vi "Button_Click.vi"(0 "Button_1":bool caption="Button 1", 5 "Button_2":bool caption="Button 2", 11 "Error_In":errorcluster) -> (15 "Error_Out":errorcluster)   [LabVIEW 2023]
doc: "This VI alternatively Clicks two boolean buttons until key down happens,"
uses:
  Controls/Click_On.ctl
panel:
  # "."
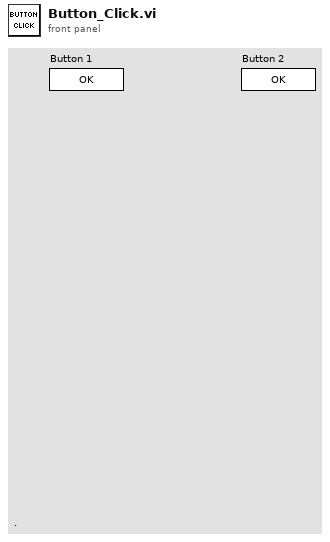
[diagram p1: front panel]
types:
  T1 = typedef "Click_On.ctl" = enum16{"Button 1", "Button 2"}
  T2 = typedef "LVRectTypeDef.ctl" = cluster{"Left":i16, "Top":i16, "Right":i16, "Bottom":i16}
  T3 = typedef "LVPositionTypeDef.ctl" = cluster{"Left":i32, "Top":i32}
  T4 = enum16{"Left Button", "Center Button", "Right Button", "Window Close"}
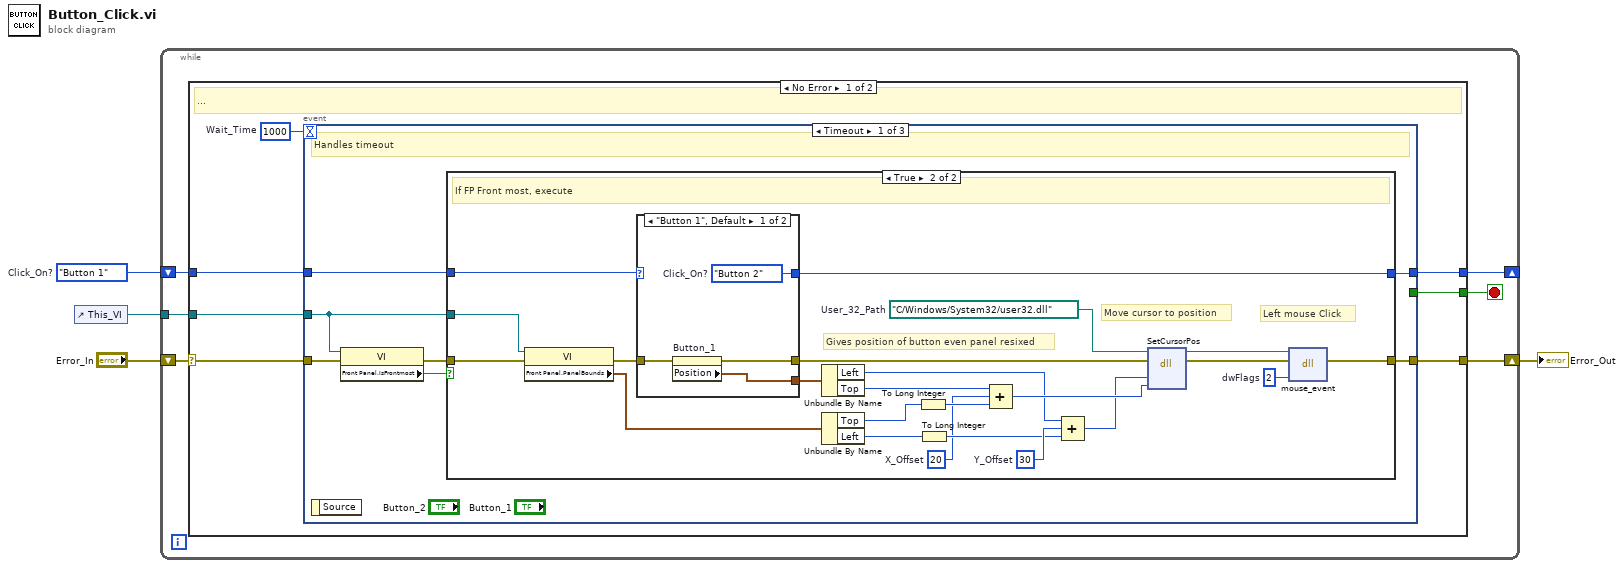
[diagram p0: block diagram]
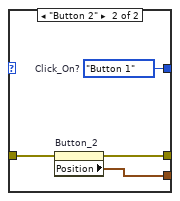
[diagram p3: hidden frame]
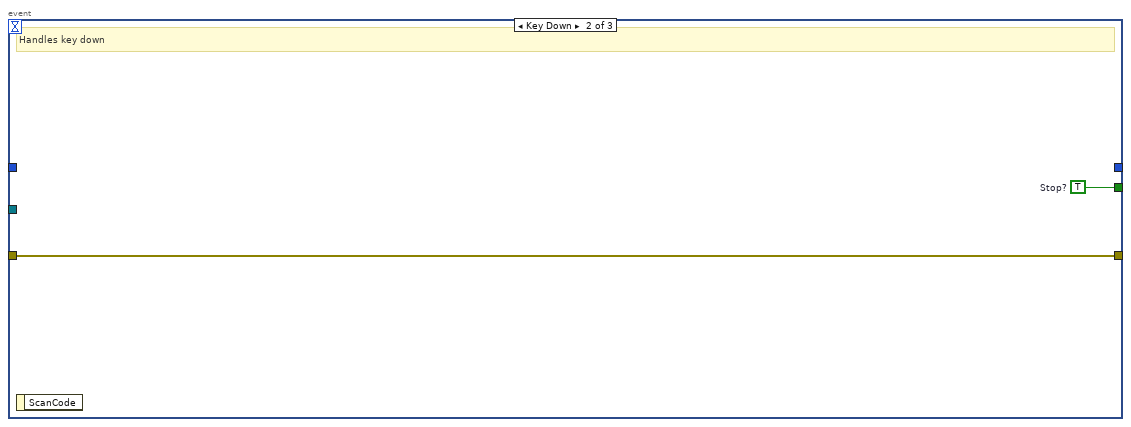
[diagram p4: hidden frame]
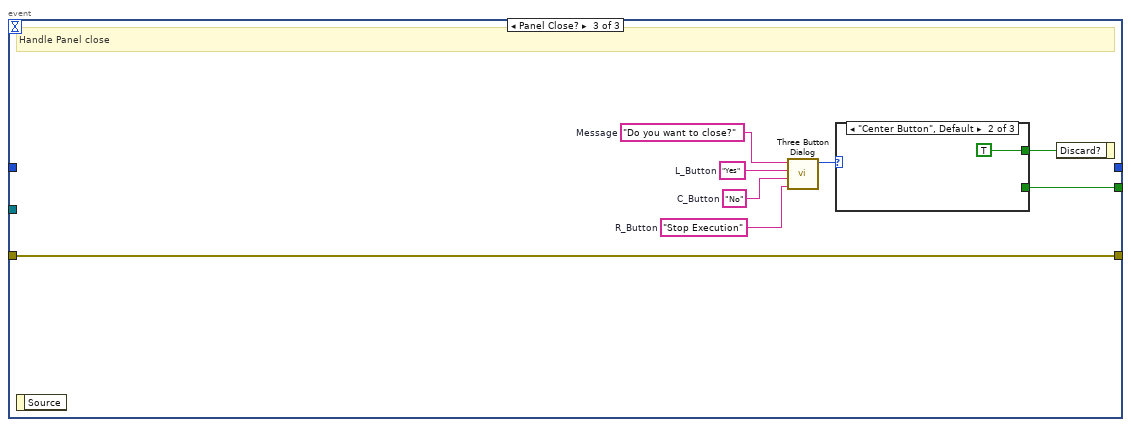
[diagram p5: hidden frame]
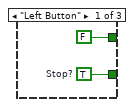
[diagram p6: hidden frame]
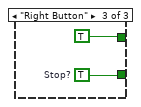
[diagram p7: hidden frame]
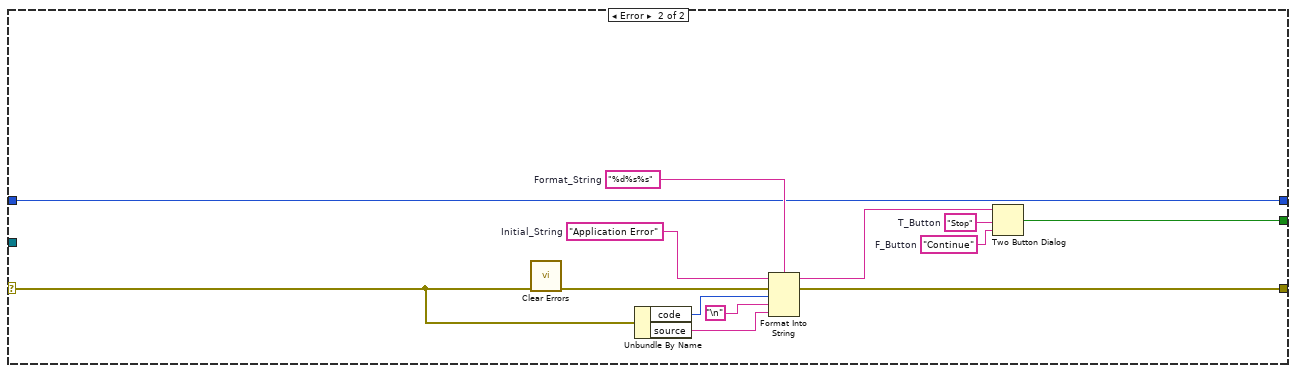
[diagram p8: hidden frame]
diagram:
  w3 = Click_On."Button 1"  # Click_On?
  n1 = control-ref of="This_VI"() -> (w1:refnum<vi>)
  n2 = while {
    shift-right: [w9] -> _
    shift-left: w3 -> [w7]
    shift-right: [w8] -> w4
    shift-left: "Error_In" -> [w10]
    tunnel: w1 -> [w5]
    stop <- w6 stop-if-true
    n3 = case shown="No Error" w10 {
      selector: w10 -> [w16 w73]
      tunnel: [w15 w74] -> w9
      tunnel: [w14 w76] -> w8
      tunnel: w7 -> [w13 w74]
      tunnel: [w12 w75] -> w6
      tunnel: w5 -> [w11 _]
      frame No Error {
        w17 = 1000  # Wait_Time
        # "..."
        n4 = event shown="[0] Timeout" {
          selector: _ -> [_ _ _]
          dyn-events: _ -> [_ _ _]
          timeout: w17 -> [_ _ _]
          tunnel: w16 -> [w21 w59 w61]
          tunnel: [w24 _ _] -> w15
          tunnel: [w22 w59 w61] -> w14
          tunnel: w13 -> [w23 _ _]
          tunnel: [_ w58 w62] -> w12
          tunnel: w11 -> [w19 _ _]
          event Timeout {
            # "Handles timeout"
            n5 = event-data() -> ()  [unwired: 1 in, 1 out]
            n6 = property class="VI"(reference=w19, error in=w21) -> (error out=w20:errorcluster, "Front Panel.IsFrontmost"=w18:bool)  [unwired: 1 out]
            n7 = case shown="True" w18 {
              tunnel: [w25 w49] -> w24
              tunnel: w23 -> [w25 w48]
              tunnel: [w26 w46] -> w22
              tunnel: w20 -> [w26 w39]
              tunnel: w19 -> [_ w30]
              frame False {
                # "If FP not front most, dont execute"
              }
              frame True {
                w28 = path "C:/Windows/System32/user32.dll"  # User_32_Path
                w45 = 2  # dwFlags
                w29 = 20  # X_Offset
                w43 = 30  # Y_Offset
                # "Gives position of button even panel resixed"
                # "Left mouse Click"
                # "Move cursor to position"
                # "If FP Front most, execute"
                n8 = property class="VI"(reference=w30, error in=w39) -> (error out=w38:errorcluster, "Front Panel.PanelBounds"=w31:T2)  [unwired: 1 out]
                n9 = case shown="\"Button 1\", Default" w48 {
                  tunnel: w38 -> [w53 w55]
                  tunnel: [w52 w57] -> w41
                  tunnel: [w51 w56] -> w40
                  tunnel: [w50 w54] -> w49
                  frame "Button 1", Default {
                    w50 = Click_On."Button 2"  # Click_On?
                    n10 = property on="Button_1" class="Bool (strict)"(error in=w53) -> (error out=w52:errorcluster, "Position"=w51:T3)  [unwired: 1 in, 1 out]
                  }
                  frame "Button 2" {
                    w54 = Click_On."Button 1"  # Click_On?
                    n11 = property on="Button_2" class="Bool (strict)"(error in=w55) -> (error out=w57:errorcluster, "Position"=w56:T3)  [unwired: 1 in, 1 out]
                  }
                }
                n12 = Unbundle By Name(w40) -> ("Left"=w37:i32, "Top"=w36:i32)
                n13 = Unbundle By Name(w31) -> ("Top"=w35:i16, "Left"=w33:i16)
                n14 = To Long Integer(number=w35) -> (32bit integer=w34:i32)
                n15 = To Long Integer(number=w33) -> (32bit integer=w32:i32)
                n16 = Compound Arithmetic op=ADD(w36, w29, w34) -> (w44:i32)
                n17 = Compound Arithmetic op=ADD(w37, w43, w32) -> (w42:i32)
                n18 = dll-call lib="?" fn="SetCursorPos"(path in=w28, error in=w41, "X_Coord"=w42, "Y_Coord"=w44) -> (path out=w27:path, error out=w47:errorcluster)  [unwired: 4 in]
                n19 = dll-call lib="?" fn="mouse_event"(path in=w27, error in=w47, "dwFlags"=w45) -> (error out=w46:errorcluster)  [unwired: 3 in, 1 out]
              }
            }
          }
          event Key Down {
            w58 = TRUE  # Stop?
            # "Handles key down"
            n20 = event-data() -> ()  [unwired: 1 in, 1 out]
          }
          event Panel Close? {
            w60 = "Stop Execution"  # R_Button
            w65 = "No"  # C_Button
            w66 = "Yes"  # L_Button
            w67 = "Do you want to close?"  # Message
            # "Handle Panel close"
            n21 = event-data() -> ()  [unwired: 1 in, 1 out]
            n22 = call <vilib>:"Three Button Dialog.vi"("Right Button Text (\"Cancel\")"=w60, "Center Button Text (\"No\")"=w65, "Left Button Text (\"Yes\")"=w66, "message"=w67) -> ("Which Button?"=w64:T4)  [unwired: 7 in]
            n23 = case shown="\"Center Button\", Default" w64 {
              tunnel: [FALSE TRUE TRUE] -> w63
              tunnel: [w68 _ w72] -> w62
              frame "Left Button" {
                w68 = TRUE  # Stop?
              }
              frame "Center Button", Default {
              }
              frame "Right Button" {
                w72 = TRUE  # Stop?
              }
            }
            n24 = event-data("Discard?"=w63) -> ()  [unwired: 1 in, 1 out]
          }
        }
      }
      frame Error {
        w81 = "%d%s%s"  # Format_String
        w82 = "Application Error"  # Initial_String
        w83 = "Stop"  # T_Button
        w84 = "Continue"  # F_Button
        n25 = call <vilib>:"Clear Errors.vi"("error in (no error)"=w73) -> ("error out"=w79:errorcluster)  [unwired: 5 in, 1 out]
        n26 = Unbundle By Name(w73) -> ("code"=w78:i32, "source"=w77:string)
        n27 = Format Into String(format string=w81, initial string=w82, error in=w79, w78, "\n", w77) -> (resulting string=w85:string, error out=w76:errorcluster)
        n28 = Two Button Dialog(message=w85, 1:w84, 2:w83) -> (T button?=w75:bool)
      }
    }
  }
  "Error_Out" <- w4
